vi "Intellifaucet_Driver.vi"(0 "VISA session":refnum<visa-resource-name>="MW100", 1 "Mode":T2=enum."Stop Flow", 2 "Semiphore":T1, 5 "Temperature(F)":dbl(slide)=58.0 scale=40.0..120.0, 7 "Percent Flow":dbl(slide)=100.0 scale=0.0..100.0, 11 "Error In":errorcluster) -> (4 "VISA session out":refnum<visa-resource-name>, 15 "Error Out":errorcluster)   [LabVIEW 2009]
uses:
  Intellfaucet Mode.ctl
  ChannelSettings.ctl
panel:
  out "created new":bool
  in  "milliseconds to wait":u32=250
  out "etime array":u32[](array[numeric])
  out "Step":i32
  out "Local?":bool
  # "%"
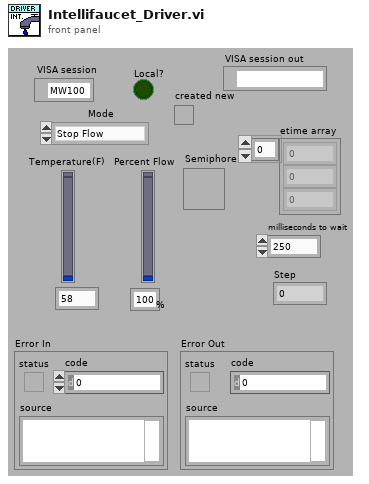
[diagram p1: front panel]
types:
  T1 = typedef "Semaphore RefNum" = refnum<k1>
  T2 = typedef "Intellfaucet Mode.ctl" = enum16{"Adjust Temp", "Adjust Flow", "Start Flow", "Stop Flow"}
  T3 = typedef "ChannelSettings.ctl" = u32
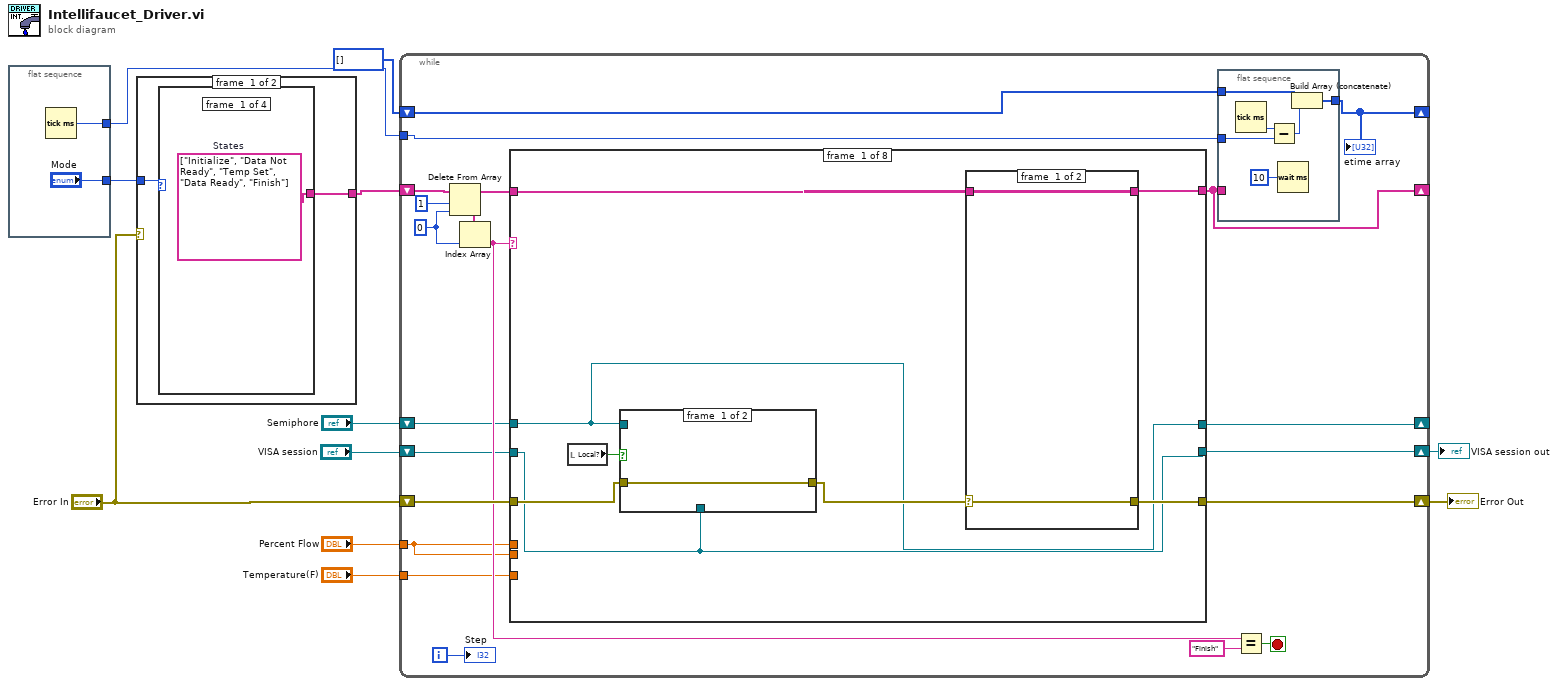
[diagram p0: block diagram]
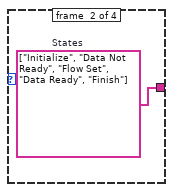
[diagram p2: hidden frame]
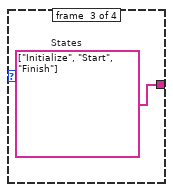
[diagram p3: hidden frame]
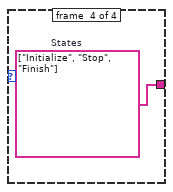
[diagram p4: hidden frame]
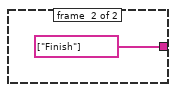
[diagram p5: hidden frame]
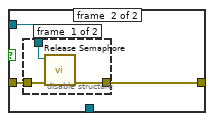
[diagram p6: hidden frame]
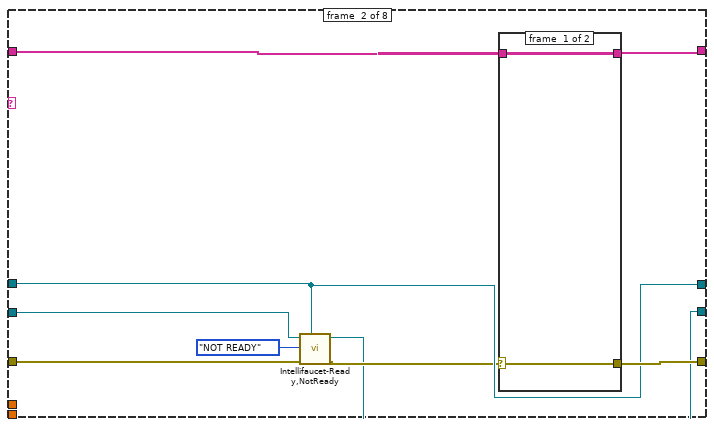
[diagram p9: hidden frame]
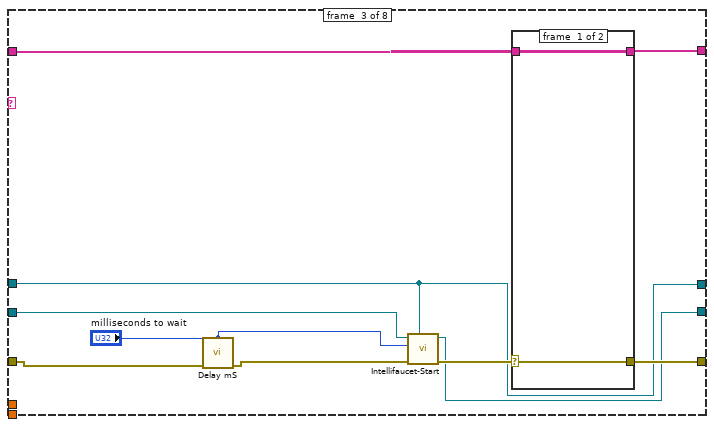
[diagram p11: hidden frame]
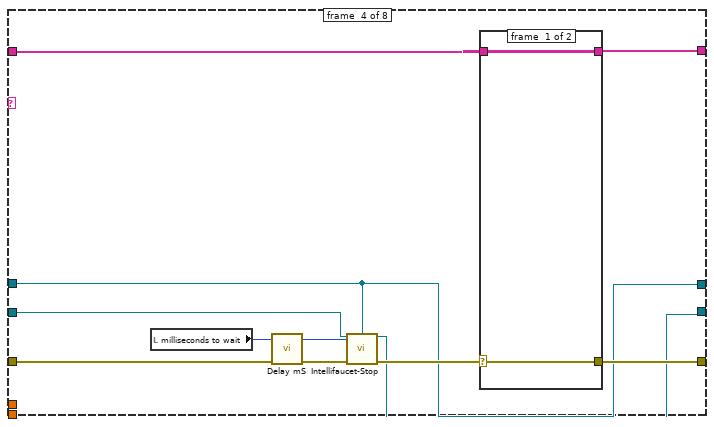
[diagram p13: hidden frame]
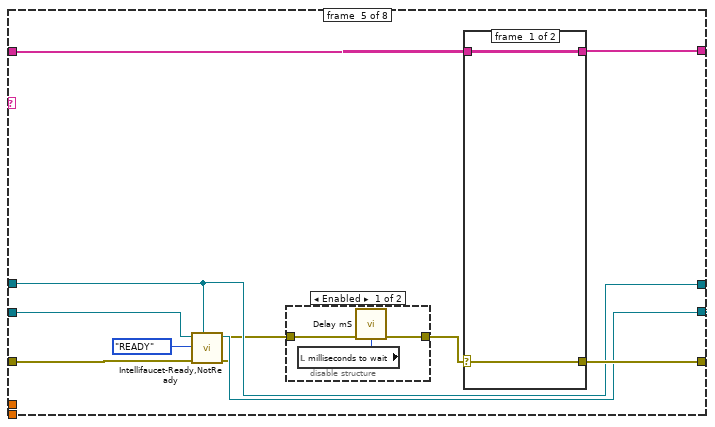
[diagram p15: hidden frame]
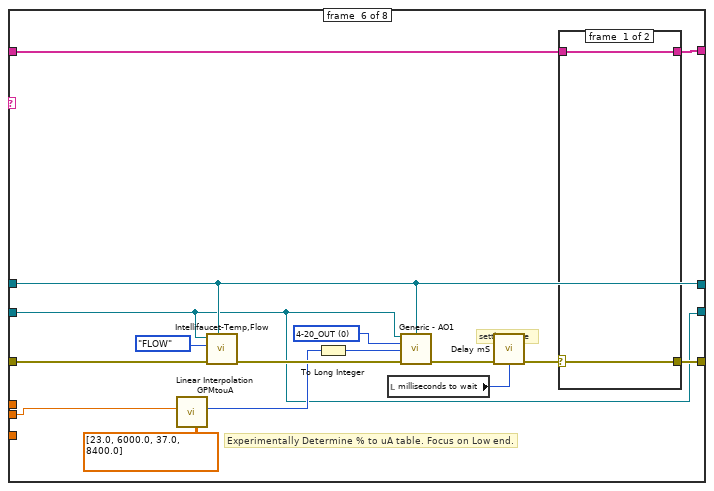
[diagram p18: hidden frame]
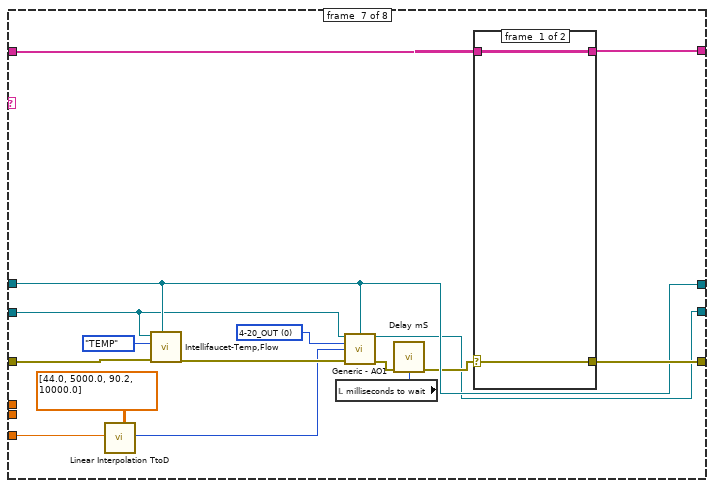
[diagram p20: hidden frame]
diagram:
  n1 = flat-sequence {
    tunnel: ["Mode"] -> w9
    tunnel: [w12] -> w4
    frame #0 {
      n2 = Tick Count (ms)() -> (millisecond timer value=w12:u32)
    }
  }
  n3 = case shown="No Error" "Error In" {
    tunnel: [w15 string[] ["Finish"] ("States")] -> w11
    tunnel: w9 -> [w14 _]
    frame #0 {
      n4 = case shown="\"Stop Flow\"" w14 {
        tunnel: [w16 w17 w18 w19] -> w15
        frame #0 {
          w16 = string[] ["Initialize", "Data Not Ready", "Temp Set", "Data Ready", "Finish"]  # States
        }
        frame #1 {
          w17 = string[] ["Initialize", "Data Not Ready", "Flow Set", "Data Ready", "Finish"]  # States
        }
        frame #2 {
          w18 = string[] ["Initialize", "Start", "Finish"]  # States
        }
        frame #3 {
          w19 = string[] ["Initialize", "Stop", "Finish"]  # States
        }
      }
    }
    frame #1 {
    }
  }
  n5 = while {
    shift-right: [w24] -> _
    shift-left: w11 -> [w41]
    shift-right: [w36] -> w10
    shift-left: "Error In" -> [w35]
    tunnel: "Percent Flow" -> [w29]
    tunnel: "Temperature(F)" -> [w30]
    shift-right: [w28] -> _
    shift-left: "Semiphore" -> [w27]
    shift-right: [w26] -> w2
    shift-left: "VISA session" -> [w31]
    tunnel: w4 -> [w22]
    shift-right: [w21] -> _
    shift-left: u32[] [] -> [w23]
    i -> [w25]
    stop <- w34 stop-if-true
    w38 = 0 ("index")
    n6 = Delete From Array(array=w41, length=1, index=w38) -> (deleted portion=w39:string[], array with subset deleted=w37:string[])
    n7 = Index Array(array=w39, index=w38) -> (element=w33:string)
    n8 = case shown="\"Initialize\"" w33 {
      tunnel: [w55 w76 w90 w104 w118 w142 w162 w177] -> w24
      tunnel: w37 -> [w54 w75 w89 w103 w117 w141 w161 w177]
      tunnel: [w53 w74 w88 w102 w116 w140 w160 w171] -> w36
      tunnel: w35 -> [w52 w73 w83 w97 w115 w139 w159 w172]
      tunnel: w31 -> [w48 w69 w85 w99 w112 w128 w151 w168]
      tunnel: w29 -> [_ _ _ _ _ _ _ _]
      tunnel: w30 -> [_ _ _ _ _ _ w153 _]
      tunnel: w29 -> [_ _ _ _ _ w133 _ _]
      tunnel: [w50 w71 w86 w100 w113 w134 w155 w170] -> w28
      tunnel: w27 -> [w50 w71 w86 w100 w113 w134 w155 w169]
      tunnel: [w48 w68 w84 w98 w111 w128 w147 w167] -> w26
      frame #0 {
        n9 = local read "Local?"() -> (w49:bool)
        n10 = case shown="True" w49 {
          tunnel: w52 -> [w56 w59]
          tunnel: [w56 w57] -> w51
          tunnel: w50 -> [_ w58]
          tunnel: w48 -> [_ _]
          frame #0 {
          }
          frame #1 {
            n11 = disable-structure shown="Enabled" {
              disable-tunnel: w59 -> [w62 w63]
              disable-tunnel: w58 -> [w61 _]
              disable-tunnel: [w60 w63] -> w57
              frame #0 {
                n12 = call <vilib>:"Release Semaphore.vi"("error in (no error)"=w62, "semaphore"=w61) -> ("error out"=w60:errorcluster)  [unwired: 4 in, 1 out]
              }
              frame #1 {
              }
            }
          }
        }
        n13 = case shown="Error" w51 {
          selector: w51 -> [w64 w66]
          tunnel: [w65 w67] -> w55
          tunnel: w54 -> [w65 w67]
          tunnel: [w64 w66] -> w53
          frame #0 {
          }
          frame #1 {
          }
        }
      }
      frame #1 {
        n14 = call "Intellifaucet-Ready,NotReady.vi"("Semiphore"=w71, "Error In"=w73, "READY?"=enum8{"READY", "NOT READY"}."NOT READY", "VISA session"=w69) -> ("Error Out"=w70:errorcluster, "dup VISA session"=w68:refnum<visa-resource-name>)  [unwired: 6 in]
        n15 = case shown="No Error" w70 {
          selector: w70 -> [w77 w79]
          tunnel: [w78 w80] -> w76
          tunnel: w75 -> [w78 w80]
          tunnel: [w77 w79] -> w74
          frame #0 {
          }
          frame #1 {
          }
        }
      }
      frame #2 {
        n16 = call "Delay mS.vi"("Error In"=w83, "milliseconds to wait"="milliseconds to wait") -> ("Error Out"=w82:errorcluster)  [unwired: 13 in]
        n17 = call "Intellifaucet-Start.vi"("Semiphore"=w86, "Error In"=w82, "mS wait"="milliseconds to wait", "VISA session"=w85) -> ("Error Out"=w87:errorcluster, "dup VISA session"=w84:refnum<visa-resource-name>)  [unwired: 6 in]
        n18 = case shown="Error" w87 {
          selector: w87 -> [w91 w93]
          tunnel: [w92 w94] -> w90
          tunnel: w89 -> [w92 w94]
          tunnel: [w91 w93] -> w88
          frame #0 {
          }
          frame #1 {
          }
        }
      }
      frame #3 {
        n19 = local read "milliseconds to wait"() -> (w95:u32)
        n20 = call "Delay mS.vi"("Error In"=w97, "milliseconds to wait"=w95) -> ("Error Out"=w96:errorcluster)  [unwired: 13 in]
        n21 = call "Intellifaucet-Stop.vi"("VISA session"=w99, "Semiphore"=w100, "mS wait"=w95, "Error In"=w96) -> ("dup VISA session"=w98:refnum<visa-resource-name>, "Error Out"=w101:errorcluster)  [unwired: 10 in]
        n22 = case shown="Error" w101 {
          selector: w101 -> [w105 w107]
          tunnel: [w106 w108] -> w104
          tunnel: w103 -> [w106 w108]
          tunnel: [w105 w107] -> w102
          frame #0 {
          }
          frame #1 {
          }
        }
      }
      frame #4 {
        n23 = call "Intellifaucet-Ready,NotReady.vi"("Semiphore"=w113, "Error In"=w115, "READY?"=enum8{"READY", "NOT READY"}."READY", "VISA session"=w112) -> ("Error Out"=w110:errorcluster, "dup VISA session"=w111:refnum<visa-resource-name>)  [unwired: 6 in]
        n24 = disable-structure shown="Enabled" {
          disable-tunnel: w110 -> [w120 w122]
          disable-tunnel: [w119 w122] -> w109
          frame #0 {
            n25 = local read "milliseconds to wait"() -> (w121:u32)
            n26 = call "Delay mS.vi"("Error In"=w120, "milliseconds to wait"=w121) -> ("Error Out"=w119:errorcluster)  [unwired: 13 in]
          }
          frame #1 {
          }
        }
        n27 = case shown="Error" w109 {
          selector: w109 -> [w123 w125]
          tunnel: [w124 w126] -> w118
          tunnel: w117 -> [w124 w126]
          tunnel: [w123 w125] -> w116
          frame #0 {
          }
          frame #1 {
          }
        }
      }
      frame #5 {
        w135 = T3 0 items=["4-20_OUT", "Pres_HI1", "Pres_HI2", "Pres_LOW", "Pres_PIN", "HEATER_TOP", "HEATER_BOT", "T_Shell", "FLOWMETER", "WATT_SENSE", "WH_TICK", "Tc_1", "Tc_2", "Tc_3", "Tc_4", "Tc_5", "Tc_6", "Tc_down", "T_Shell_2", "T_Shell_3", "T_Shell_4", "RTD_IN", "RTD_OUT", "RTD_AMB", "INTF_TEMPFLO", "INTF_READY", "INTF_START", "INTF_STOP", "DRM_LOW", "DRM_HIGH", "PWR_MAIN", "VLV_DUMP", "VLV_OUT", "VLV_IN", "WATT_HOURS", "FLOW(SAMPLE)", "GALLONS", "FLOW(GPM)"] ("Channel_Enum")
        # "Experimentally Determine % to uA table. Focus on Low end."
        # "settling time"
        n28 = call "Linear Interpolation GPMtouA.vi"("2D Flow Data (GPM,uA)"=dbl[][] [[23.0, 6000.0], [37.0, 8400.0]] ("Interpolation Table(Xs,Ys)"), "GPM Target"=w133) -> ("uA Output"=w132:i32)  [unwired: 9 in]
        n29 = call "Intellifaucet-Temp,Flow.vi"("Semiphore"=w134, "Error In"=w139, "TEMP,FLOW"=enum8{"TEMP", "FLOW"}."FLOW", "VISA session"=w128) -> ("Error Out"=w137:errorcluster)  [unwired: 6 in, 1 out]
        n30 = To Long Integer(number=w132) -> (32bit integer=w136:i32)
        n31 = local read "milliseconds to wait"() -> (w127:u32)
        n32 = call "Generic - AO1.vi"("VISA session"=w128, "Semiphore"=w134, "Channel_Enum"=w135, "Output Value (0)"=w136, "Error In"=w137) -> ("error out"=w130:errorcluster)  [unwired: 9 in, 1 out]
        n33 = call "Delay mS.vi"("Error In"=w130, "milliseconds to wait"=w127) -> ("Error Out"=w129:errorcluster)  [unwired: 13 in]
        n34 = case shown="Error" w129 {
          selector: w129 -> [w143 w145]
          tunnel: [w144 w146] -> w142
          tunnel: w141 -> [w144 w146]
          tunnel: [w143 w145] -> w140
          frame #0 {
          }
          frame #1 {
          }
        }
      }
      frame #6 {
        w156 = T3 0 items=["4-20_OUT", "Pres_HI1", "Pres_HI2", "Pres_LOW", "Pres_PIN", "HEATER_TOP", "HEATER_BOT", "T_Shell", "FLOWMETER", "WATT_SENSE", "WH_TICK", "Tc_1", "Tc_2", "Tc_3", "Tc_4", "Tc_5", "Tc_6", "Tc_down", "T_Shell_2", "T_Shell_3", "T_Shell_4", "RTD_IN", "RTD_OUT", "RTD_AMB", "INTF_TEMPFLO", "INTF_READY", "INTF_START", "INTF_STOP", "DRM_LOW", "DRM_HIGH", "PWR_MAIN", "VLV_DUMP", "VLV_OUT", "VLV_IN", "WATT_HOURS", "FLOW(SAMPLE)", "GALLONS", "FLOW(GPM)"] ("Channel_Enum")
        n35 = call "Linear Interpolation TtoD.vi"("Interpolation Table(Xs,Ys)"=dbl[][] [[44.0, 5000.0], [90.2, 10000.0]], "Interp. X"=w153) -> ("Output Y"=w154:i32)  [unwired: 9 in]
        n36 = call "Intellifaucet-Temp,Flow.vi"("Semiphore"=w155, "Error In"=w159, "TEMP,FLOW"=enum8{"TEMP", "FLOW"}."TEMP", "VISA session"=w151) -> ("Error Out"=w157:errorcluster)  [unwired: 6 in, 1 out]
        n37 = local read "milliseconds to wait"() -> (w150:u32)
        n38 = call "Generic - AO1.vi"("VISA session"=w151, "Semiphore"=w155, "Channel_Enum"=w156, "Output Value (0)"=w154, "Error In"=w157) -> ("dup VISA session"=w147:refnum<visa-resource-name>, "error out"=w149:errorcluster)  [unwired: 9 in]
        n39 = call "Delay mS.vi"("Error In"=w149, "milliseconds to wait"=w150) -> ("Error Out"=w148:errorcluster)  [unwired: 13 in]
        n40 = case shown="Error" w148 {
          selector: w148 -> [w163 w165]
          tunnel: [w164 w166] -> w162
          tunnel: w161 -> [w164 w166]
          tunnel: [w163 w165] -> w160
          frame #0 {
          }
          frame #1 {
          }
        }
      }
      frame #7 {
        n41 = Call Chain() -> (call chain=w173:string[])
        n42 = Array Size(array=w173) -> (size(s)=w174:i32)
        n43 = Equal?(x=w174, y=1) -> (x = y?=w176:bool)
        "Local?" <- w176
        n44 = case shown="True" w176 {
          tunnel: [w179 w181] -> w170
          tunnel: w172 -> [w180 w194]
          tunnel: [w180 w187] -> w171
          tunnel: w169 -> [w179 _]
          tunnel: w168 -> [w178 w183]
          tunnel: [w178 w186] -> w167
          frame #0 {
          }
          frame #1 {
            n45 = call <vilib>:"Obtain Semaphore Reference.vi"("error in (no error)"=w194, "size (1)"=1) -> ("error out"=w185:errorcluster, "created new"=→"created new":bool, "semaphore"=w181:T1)  [unwired: 3 in]
            n46 = call "YKMW100 Close.vi"("VISA session"=w183, "error in (no error)"=w185) -> ("error out"=w184:errorcluster)  [unwired: 13 in]
            n47 = local write "Semiphore"(w181) -> ()
            n48 = call "YKMW100 Initialize.vi"("VISA session (TCPIP::)"=w183, "error in (no error)"=w184) -> ("dup VISA session"=w188:refnum<visa-resource-name>, "error out"=w191:errorcluster)  [unwired: 12 in]
            n49 = property class="Instr"(reference=w188, error in=w191, "General Settings:Timeout Value"=u32 2000) -> (reference out=w189:refnum<visa-resource-name>, error out=w190:errorcluster)
            n50 = call "YKMW100 Mode Control.vi"("VISA session"=w189, "Model"=enum16{"Meausurement Mode", "Setting Mode"}."Meausurement Mode", "error in (no error)"=w190) -> ("dup VISA session"=w186:refnum<visa-resource-name>, "error out"=w187:errorcluster)  [unwired: 11 in]
          }
        }
      }
    }
    n51 = flat-sequence {
      tunnel: w24 -> [_]
      tunnel: [w44] -> w21
      tunnel: w23 -> [w43]
      tunnel: w22 -> [w42]
      frame #0 {
        n52 = Tick Count (ms)() -> (millisecond timer value=w45:u32)
        n53 = Subtract(x=w45, y=w42) -> (x-y=w46:u32)
        n54 = Wait (ms)(milliseconds to wait=u32 10) -> ()  [unwired: 1 out]
        n55 = Build Array (concatenate)(w43, w46) -> (w44:u32[])
      }
    }
    n56 = Equal?(x=w33, y="Finish") -> (x = y?=w34:bool)
    "Step" <- w25
    "etime array" <- w21
  }
  "Error Out" <- w10
  "VISA session out" <- w2
